vi "Square_Pulse.vi"() -> ()   [LabVIEW 2016]
panel:
  out "Voltage Out":dbl
  out "unsigned 16-bit out":u16
  in  "High Voltage (V)":dbl
  in  "Time":dbl
  in  "High Voltage Width (us)":dbl
  in  "Pulse Center (us)":dbl
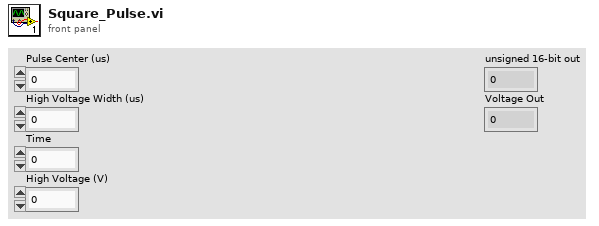
[diagram p1: front panel]
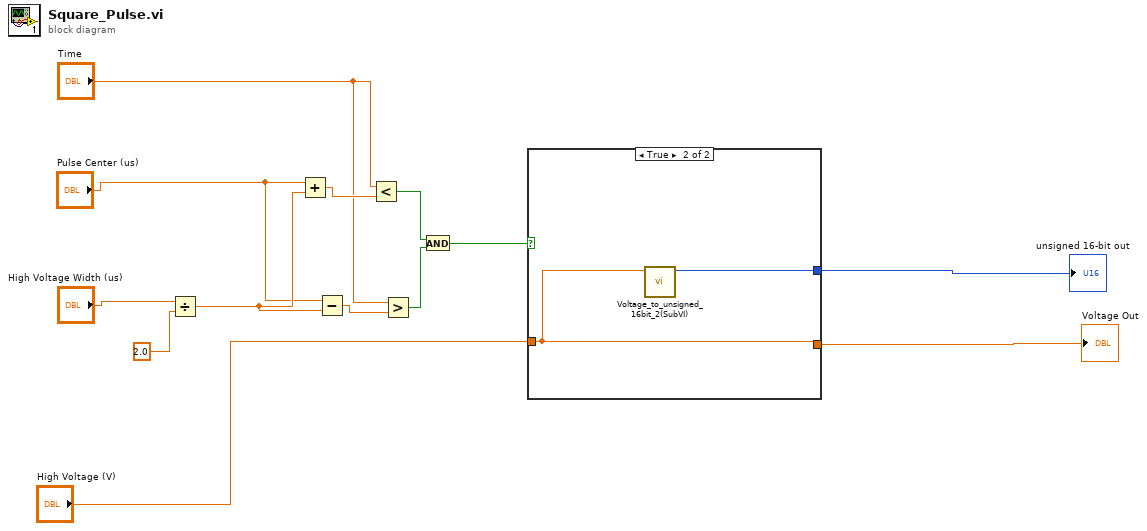
[diagram p0: block diagram]
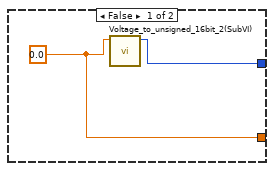
[diagram p2: hidden frame]
diagram:
  n1 = Divide(x="High Voltage Width (us)", y=2.0) -> (x/y=w11:dbl)
  n2 = Add(x="Pulse Center (us)", y=w11) -> (x+y=w10:dbl)
  n3 = Subtract(x="Pulse Center (us)", y=w11) -> (x-y=w8:dbl)
  n4 = Less?(x="Time", y=w10) -> (x < y?=w6:bool)
  n5 = Greater?(x="Time", y=w8) -> (0:w5:bool)
  n6 = And(x=w6, y=w5) -> (x .and. y?=w4:bool)
  n7 = case shown="True" w4 {
    tunnel: "High Voltage (V)" -> [_ w16]
    tunnel: [w15 w17] -> w2
    tunnel: [w14 w16] -> w1
    frame False {
      w14 = 0.0
      n8 = call "Voltage_to_unsigned_16bit_2(SubVI).vi"("Voltage_in"=w14) -> ("unsigned 16bit integer"=w15:u16)  [unwired: 10 in]
    }
    frame True {
      n9 = call "Voltage_to_unsigned_16bit_2(SubVI).vi"("Voltage_in"=w16) -> ("unsigned 16bit integer"=w17:u16)  [unwired: 10 in]
    }
  }
  "unsigned 16-bit out" <- w2
  "Voltage Out" <- w1
